vi "index_normal_curve.vi"(0 "y1":dbl, 2 "Media":dbl, 5 "y2":dbl, 7 "y3":dbl, 9 "y4":dbl, 11 "error in (no error)":errorcluster) -> (4 "max":dbl, 6 "min":dbl, 15 "error out":errorcluster)   [LabVIEW 2019]
panel:
  in  "Tab Control":enum32{"Page 1", "Page 2"}(tab)
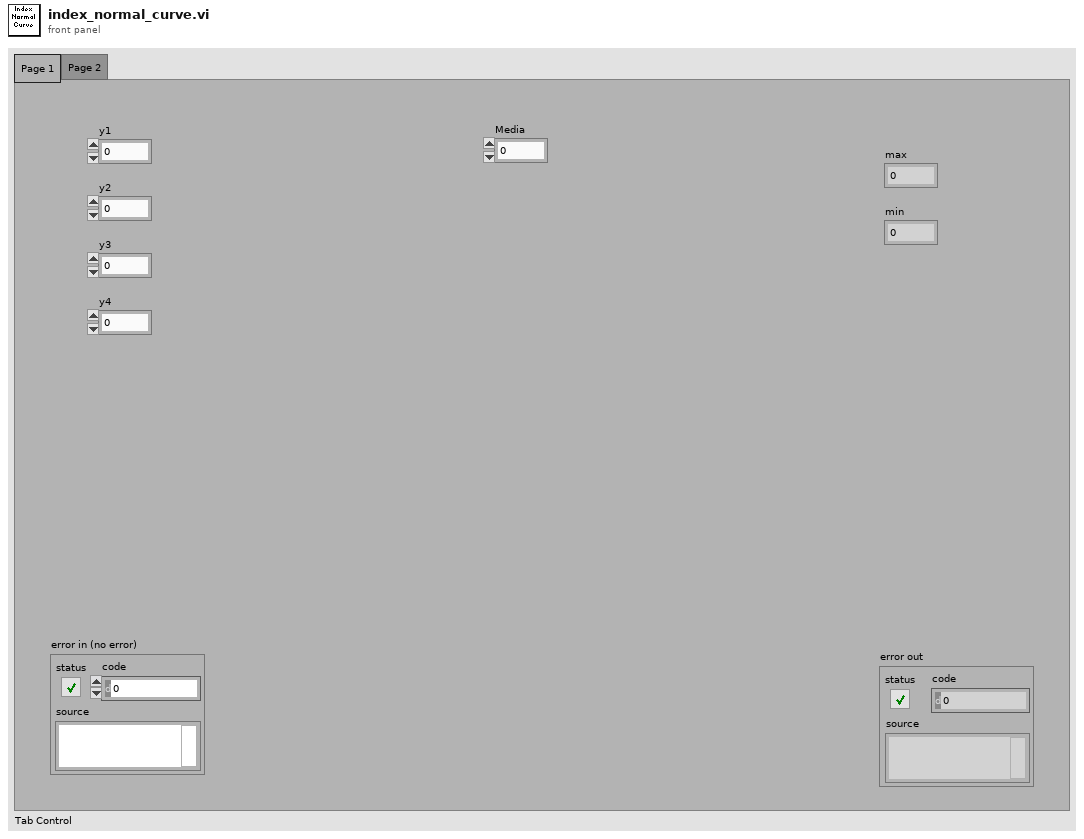
[diagram p1: front panel]
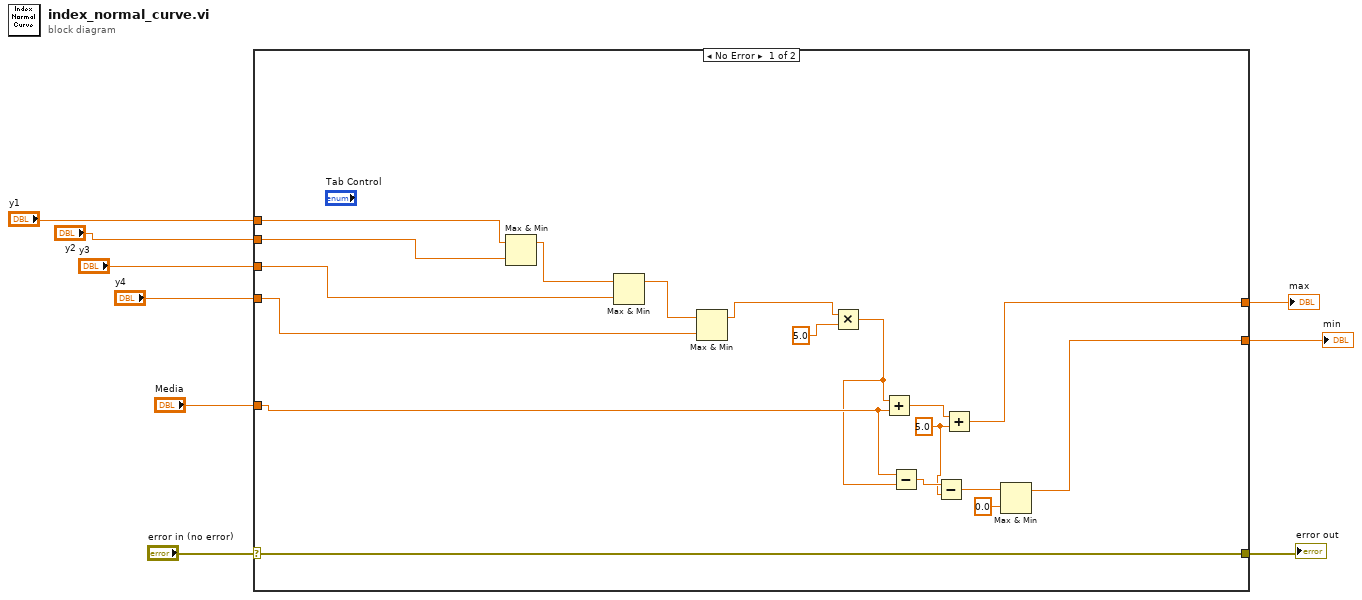
[diagram p0: block diagram]
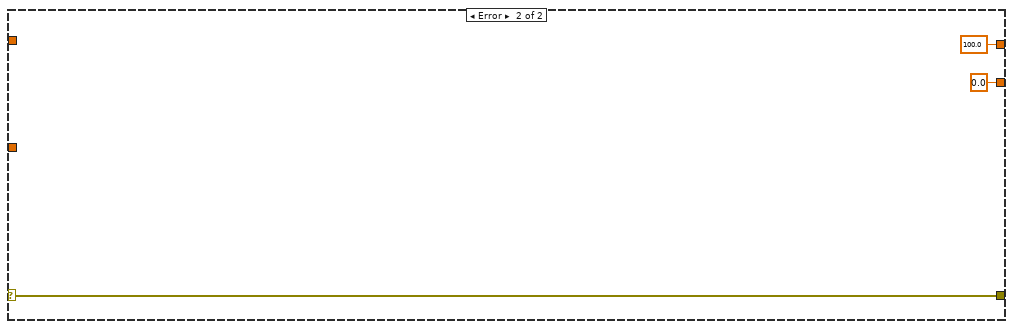
[diagram p2: hidden frame]
diagram:
  n1 = case shown="No Error" "error in (no error)" {
    selector: "error in (no error)" -> [w25 w30]
    tunnel: [w25 w30] -> w8
    tunnel: "y4" -> [w24 _]
    tunnel: "y3" -> [w23 _]
    tunnel: "y1" -> [w22 _]
    tunnel: "y2" -> [w21 _]
    tunnel: [w13 0.0] -> w3
    tunnel: [w19 100.0] -> w2
    tunnel: "Media" -> [w18 _]
    frame No Error {
      w16 = 5.0 ("y")
      n2 = Max & Min(x=w22, y=w21) -> (max(x,y)=w26:dbl)  [unwired: 1 out]
      n3 = Max & Min(x=w26, y=w23) -> (max(x,y)=w27:dbl)  [unwired: 1 out]
      n4 = Max & Min(x=w27, y=w24) -> (max(x,y)=w11:dbl)  [unwired: 1 out]
      n5 = Multiply(x=w11, y=5.0) -> (x*y=w10:dbl)
      n6 = Add(x=w10, y=w18) -> (x+y=w20:dbl)
      n7 = Subtract(x=w18, y=w10) -> (x-y=w17:dbl)
      n8 = Subtract(x=w17, y=w16) -> (x-y=w15:dbl)
      n9 = Add(x=w20, y=w16) -> (x+y=w19:dbl)
      n10 = Max & Min(x=w15, y=0.0) -> (max(x,y)=w13:dbl)  [unwired: 1 out]
    }
    frame Error {
    }
  }
  "error out" <- w8
  "max" <- w2
  "min" <- w3
